vi "AWG Calculate and Set Gain&Offset by AmpX.vi"(6 "Pins":string[](array[string]), 7 "AmpGain":i32=1, 8 "error in":errorcluster, 9 "VLo":dbl format="%#_13g", 10 "VHi":dbl format="%#_13g", 11 "Semiconductor Module Context In":T1) -> (0 "error out":errorcluster, 2 "Offset":dbl, 3 "Gain":dbl)   [LabVIEW 2013]
uses:
  <vilib>/NI_TestStand_SemiconductorModule/NI_TestStand_Semiconductor_Module.lvlibp/PinMap/General/SemiconductorModuleContext.ctl
  <vilib>/NI_TestStand_SemiconductorModule/NI_TestStand_Semiconductor_Module.lvlibp
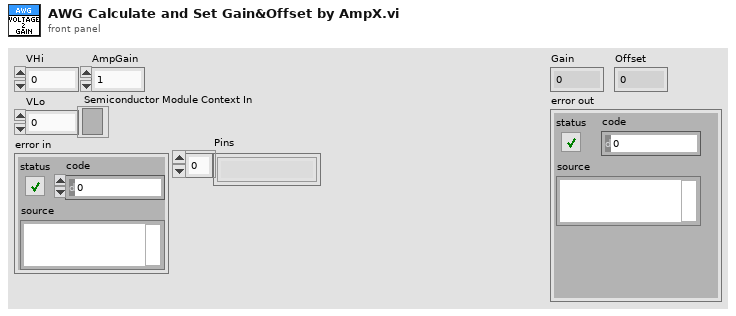
[diagram p1: front panel]
types:
  T1 = typedef "NI_TestStand_Semiconductor_Module.lvlibp/SemiconductorModuleContext.ctl" = refnum<k7>
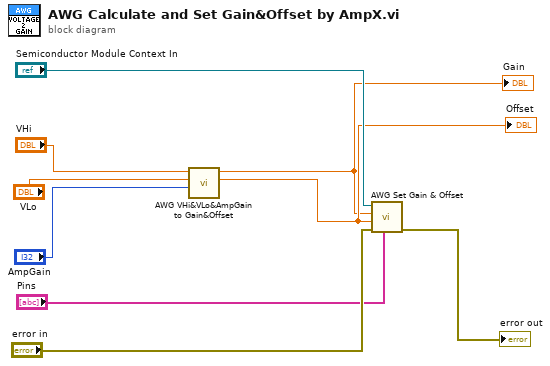
[diagram p0: block diagram]
diagram:
  n1 = call "AWG VHi&VLo&AmpGain to Gain&Offset.vi"("AmpGain"="AmpGain", "VLo"="VLo", "VHi"="VHi") -> ("Offset"=w2:dbl, "Gain"=w1:dbl)  [unwired: 7 in]
  "Gain" <- w1
  "Offset" <- w2
  n2 = call "AWG Set Gain & Offset.vi"("Pins"="Pins", "error in"="error in", "Offset"=w2, "Gain"=w1, "Semiconductor Module Context In"="Semiconductor Module Context In") -> ("error out"=→"error out":errorcluster)  [unwired: 4 in, 2 out]
